vi "Launcher.vi"   [LabVIEW 2023, in "Example Iterator NR Actor Auto Iteration Notification.lvlib"]
doc: "Launches the Example Actor that shows the operation of the Iterator Actor framework."
uses:
  Example Iterator NR Actor Auto Iteration Notification.lvlib
  Example Actor/Example Actor.lvclass
  <vilib>/ActorFramework/Actor/Actor.lvclass
panel:
  # "Launch this VI to start the example"
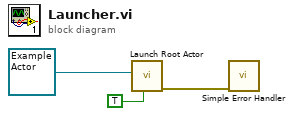
[diagram p0: block diagram]
diagram:
  n1 = call <vilib>:"Launch Root Actor.vi"("Open Actor Core front panel? (F)"=TRUE, "Actor"=refnum<class "Example Actor.lvclass"> refnum ("Example Iterator NR Actor Auto Iteration Notification.lvlib:Example Actor.lvclass")) -> ("error out"=w3:errorcluster)  [unwired: 8 in, 1 out]
  n2 = call <vilib>:"Simple Error Handler.vi"("error in (no error)"=w3) -> ()  [unwired: 4 in, 5 out]
